vi "[Test] File or directory exists.vi"() -> ()   [LabVIEW 2015, in "Tests.lvlib"]
uses:
  Tests.lvlib
  Protocol.ctl
  classes/File Transfer Behavior/Type.ctl
  classes/File Transfer Behavior/File Transfer Behavior.lvclass
panel:
  out "Type":T1
  out "Exists?":bool
  in  "Password":string
  in  "Username":string
  in  "Protocol":T2
  in  "Address":string
  in  "Path":string
  out "error out":errorcluster
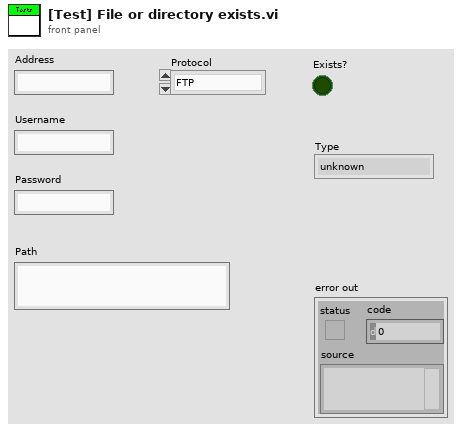
[diagram p1: front panel]
types:
  T1 = typedef "RT Management.lvlib/File Transfer Behavior.lvclass/Type.ctl" = enum16{"unknown", "file", "directory"}
  T2 = typedef "Tests.lvlib/Protocol.ctl" = enum16{"FTP", "WebDAV"}
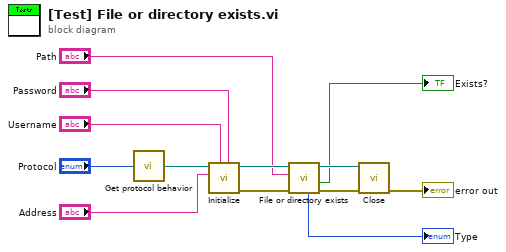
[diagram p0: block diagram]
diagram:
  n1 = call "Get protocol behavior.vi"("Protocol"="Protocol") -> ("RT Management.lvlib:FTP.lvclass"=w13:refnum<class "File Transfer Behavior.lvclass">)
  n2 = call-dynamic "Initialize.vi"("Password"="Password", "Username"="Username", "Address"="Address", "File Transfer Behavior in"=w13) -> ("error out"=w12:errorcluster, "File Transfer Behavior out"=w11:refnum<class "File Transfer Behavior.lvclass">)  [unwired: 6 in]
  n3 = call-dynamic "File or directory exists.vi"("error in (no error)"=w12, "Path"="Path", "File Transfer Behavior in"=w11) -> ("error out"=w10:errorcluster, "Exists?"=→"Exists?":bool, "File Transfer Behavior out"=w9:refnum<class "File Transfer Behavior.lvclass">, "Type"=→"Type":T1)  [unwired: 4 in, 1 out]
  n4 = call-dynamic "Close.vi"("error in (no error)"=w10, "File Transfer Behavior in"=w9) -> ("error out"=→"error out":errorcluster)  [unwired: 9 in]
